vi "tax list.vi"(10 "Parren VI":refnum<vi>) -> ()   [LabVIEW 2016, in "Tax_calculation.lvclass"]
uses:
  Tax_calculation.lvclass
  xControl_Table/builds/ZebraTable.lvlibp/XControl 1.xctl
panel:
  in  "XControl 1":string[][](xcontrol)
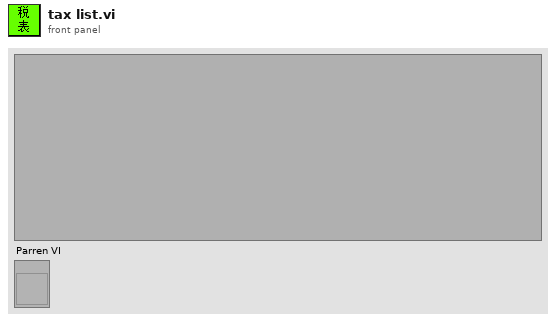
[diagram p1: front panel]
types:
  T1 = typedef "LVRectTypeDef.ctl" = cluster{"Left":i16, "Top":i16, "Right":i16, "Bottom":i16}
  T2 = enum32{"Invalid", "Standard", "Closed", "Hidden", "Minimized", "Maximized"}
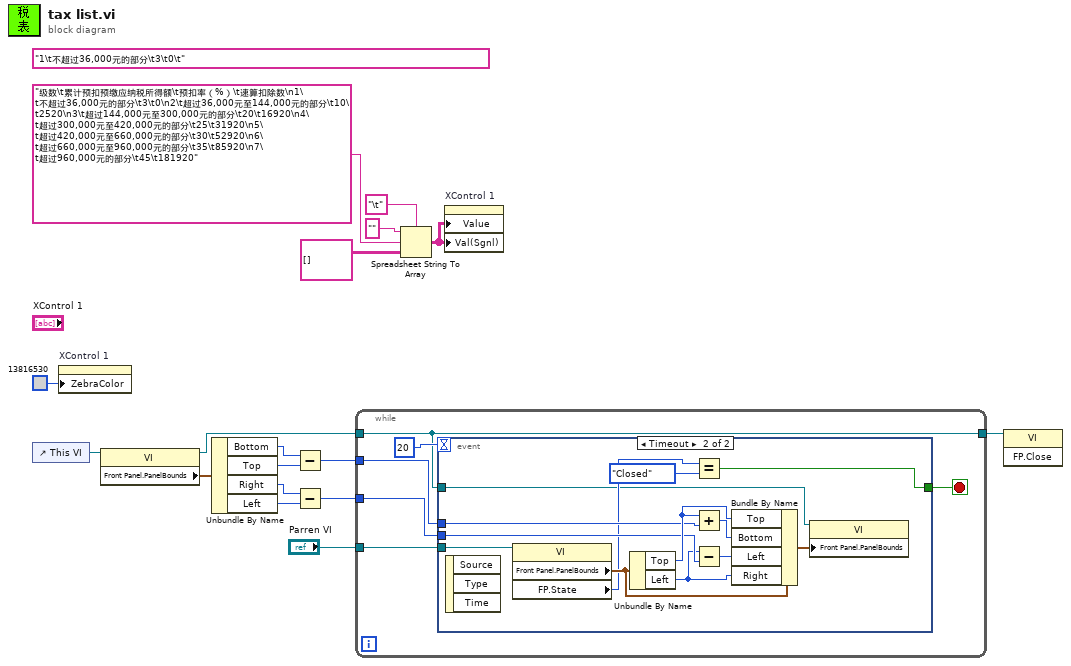
[diagram p0: block diagram]
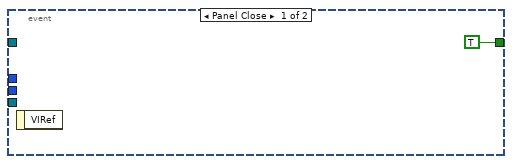
[diagram p2: hidden frame]
diagram:
  (unwired) "1\t不超过36,000元的部分\t3\t0\t"
  n1 = control-ref of="This VI"() -> (w7:refnum<vi>)
  n2 = property on="XControl 1" class="XControl 1 (strict)"("ZebraColor"=u32 13816530) -> ()  [unwired: 2 in, 2 out]
  n3 = property class="VI"(reference=w7) -> (reference out=w2:refnum<vi>, "Front Panel.PanelBounds"=w8:T1)  [unwired: 1 in, 1 out]
  n4 = Unbundle By Name(w8) -> ("Bottom"=w10:i16, "Top"=w9:i16, "Right"=w6:i16, "Left"=w5:i16)
  n5 = Subtract(x=w10, y=w9) -> (x-y=w3:i16)
  n6 = Subtract(x=w6, y=w5) -> (x-y=w4:i16)
  n7 = while {
    tunnel: "Parren VI" -> [w22]
    tunnel: w4 -> [w20]
    tunnel: w3 -> [w19]
    tunnel: w2 -> [w18]
    tunnel: [w18] -> w1
    stop <- w21 stop-if-true
    n8 = event shown="[1] Timeout" {
      selector: _ -> [_ _]
      dyn-events: _ -> [_ _]
      timeout: 20 -> [_ _]
      tunnel: w22 -> [_ w37]
      tunnel: [TRUE w25] -> w21
      tunnel: w20 -> [_ w33]
      tunnel: w19 -> [_ w32]
      tunnel: w18 -> [_ w27]
      event Panel Close {
        n9 = event-data() -> ()  [unwired: 1 in, 1 out]
      }
      event Timeout {
        n10 = event-data() -> ()  [unwired: 1 in, 3 out]
        n11 = property class="VI"(reference=w37) -> ("Front Panel.PanelBounds"=w34:T1, "FP.State"=w30:T2)  [unwired: 1 in, 2 out]
        n12 = Unbundle By Name(w34) -> ("Top"=w35:i16, "Left"=w26:i16)
        n13 = Equal?(x=w30, y=T2."Closed") -> (x = y?=w25:bool)
        n14 = Add(x=w35, y=w32) -> (x+y=w36:i16)
        n15 = Subtract(x=w26, y=w33) -> (x-y=w31:i16)
        n16 = Bundle By Name(cluster=w34, "Top"=w35, "Bottom"=w36, "Left"=w31, "Right"=w26) -> (w28:T1)
        n17 = property class="VI"(reference=w27, "Front Panel.PanelBounds"=w28) -> ()  [unwired: 1 in, 2 out]
      }
    }
  }
  n18 = Spreadsheet String To Array(delimiter (Tab)="\t", format string="", spreadsheet string="级数\t累计预扣预缴应纳税所得额\t预扣率（%）\t速算扣除数\n1\t不超过36,000元的部分\t3\t0\n2\t超过36,000元至144,000元的部分\t10\t2520\n3\t超过144,000元至300,000元的部分\t20\t16920\n4\t超过300,000元至420,000元的部分\t25\t31920\n5\t超过420,000元至660,000元的部分\t30\t52920\n6\t超过660,000元至960,000元的部分\t35\t85920\n7\t超过960,000元的部分\t45\t181920", array type (2D Dbl)=string[][] [] ("XControl 1")) -> (array=w12:string[][])
  n19 = property on="XControl 1" class="XControl 1 (strict)"("Value"=w12, "Val(Sgnl)"=w12) -> ()  [unwired: 2 in, 2 out]
  n20 = invoke class="VI" method="FP.Close"(reference=w1) -> ()  [unwired: 2 in, 3 out]
